vi "CRC-16.vi"(9 "string_hex":string="\u0001\u0003\u0000\u0001\u0000\u0002") -> (10 "string&CRC-16":string)   [LabVIEW 2017]
panel:
  out "CRC":string
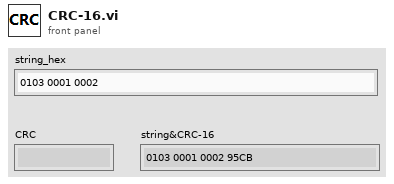
[diagram p1: front panel]
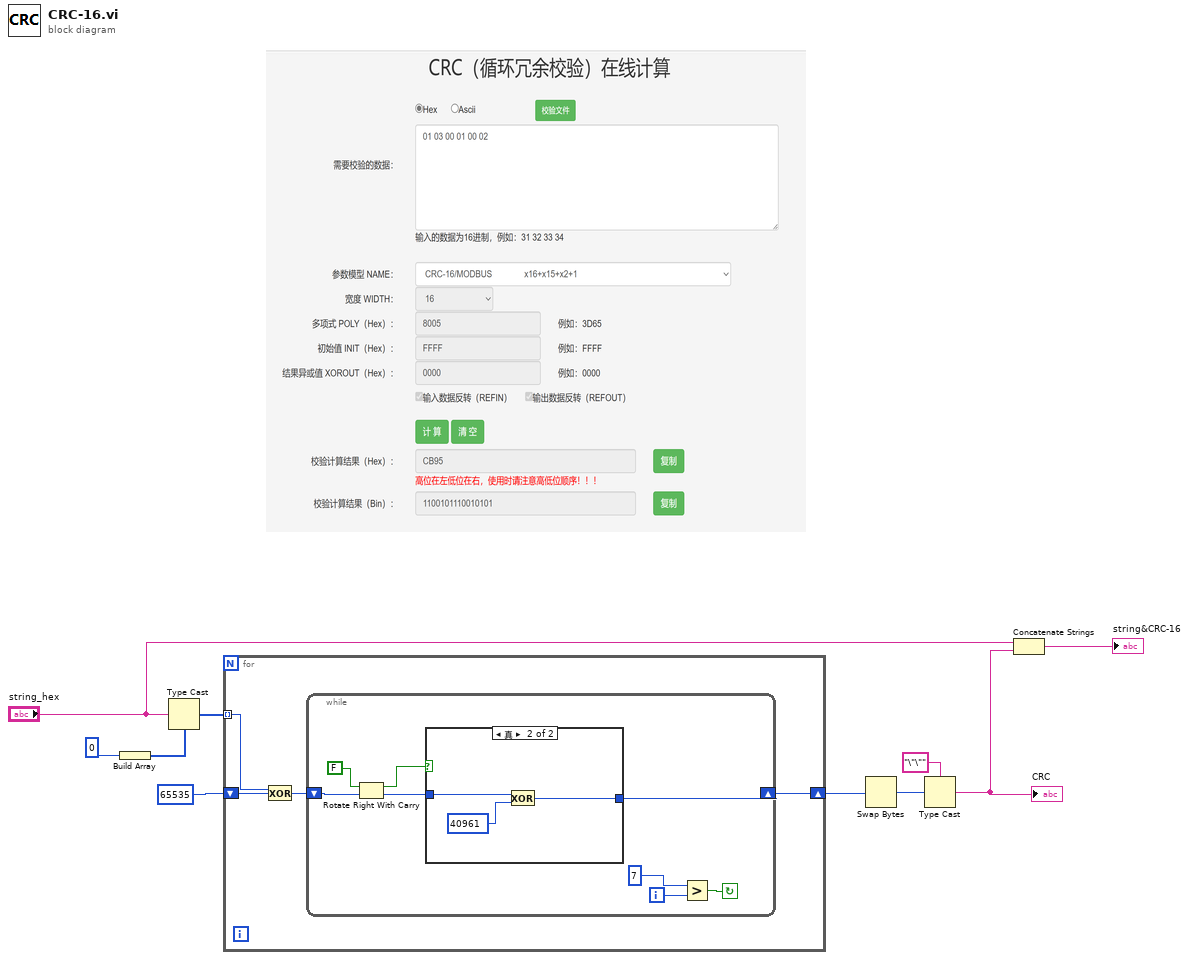
[diagram p0: block diagram]
diagram:
  n1 = Build Array(u8 0) -> (w9:u8[])
  n2 = Type Cast(type=w9, x="string_hex") -> (*(type *) &x=w7:u8[])
  n3 = for {
    tunnel: w7 -> [w12] mode=indexing
    shift-right: [w13] -> w6
    shift-left: u16 65535 -> [w11]
    n4 = Exclusive Or(1:w11, 2:w12) -> (0:w14:u16)
    n5 = while {
      shift-right: [w22] -> w13
      shift-left: w14 -> [w17]
      i -> [w21]
      stop <- w19 continue-if-true
      n6 = Rotate Right With Carry(2:w17, 3:FALSE ("进位")) -> (0:w15:u16, 1:w16:bool)
      n7 = case shown="真" w16 {
        tunnel: w15 -> [w23 w26]
        tunnel: [w23 w24] -> w22
        frame False {
        }
        frame True {
          n8 = Exclusive Or(1:u16 40961, 2:w26) -> (0:w24:u16)
        }
      }
      n9 = Greater?(x=7, y=w21) -> (0:w19:bool)
    }
  }
  n10 = Swap Bytes(anything=w6) -> (byte swapped=w5:u16)
  n11 = Type Cast(type="\"\"" ("类型"), x=w5) -> (*(type *) &x=w2:string)
  "CRC" <- w2
  n12 = Concatenate Strings("string_hex", w2) -> (→"string&CRC-16":string)
